vi "align set.vi"(8 "error in (no error)":errorcluster, 11 "align position":T1) -> (0 "error out":errorcluster, 1 "position out":cluster{"X":dbl, "y":dbl, "degree":dbl})   [LabVIEW 2019]
uses:
  align position.ctl
  subVI/move/position cluster.ctl
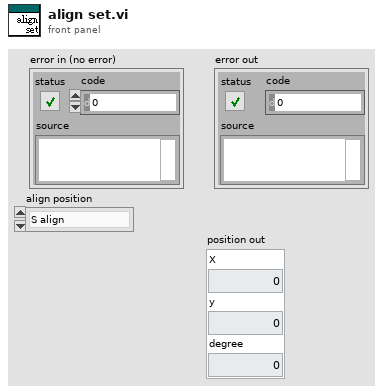
[diagram p1: front panel]
types:
  T1 = typedef "align position.ctl" = enum16{"S align", "vision align", "box align", "box to room align"}
  T2 = typedef "position cluster.ctl" = cluster{"X":dbl, "Y":dbl, "Angle":dbl}
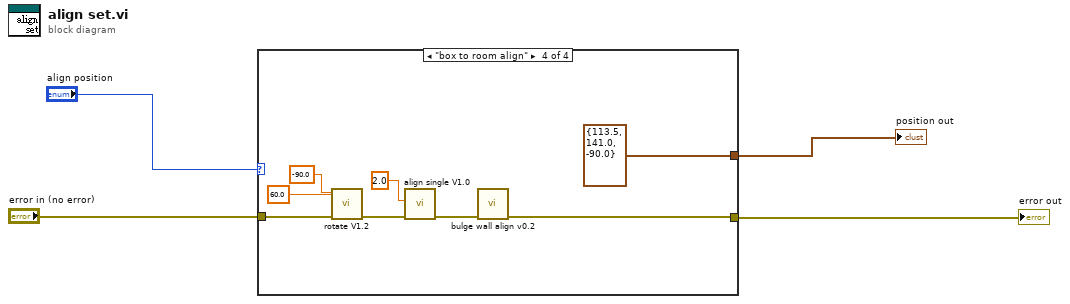
[diagram p0: block diagram]
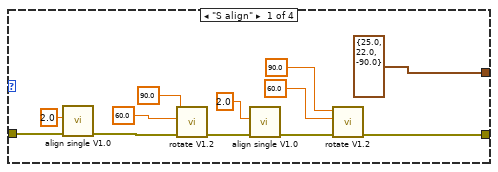
[diagram p2: hidden frame]
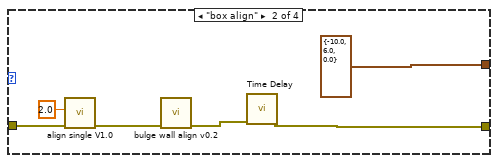
[diagram p3: hidden frame]
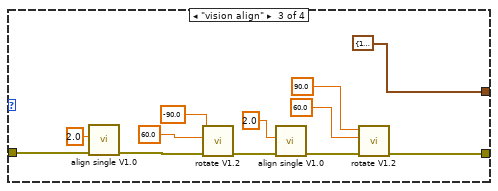
[diagram p4: hidden frame]
diagram:
  n1 = case shown="\"box to room align\"" "align position" {
    tunnel: "error in (no error)" -> [w16 w20 w25 w40]
    tunnel: [w15 w17 w24 w35] -> w3
    tunnel: [cluster{"x":dbl, "y":dbl, "degree":dbl} {"x"=25.0, "y"=22.0, "degree"=-90.0} ("position out") T2 {"X"=-10.0, "Y"=6.0, "Angle"=0.0} ("position out") cluster{"x":dbl, "y":dbl, "degree":dbl} {"x"=103.0, "y"=178.0, "degree"=0.0} ("position out") T2 {"X"=113.5, "Y"=141.0, "Angle"=-90.0} ("position out")] -> w1
    frame "S align" {
      n2 = call "align single V1.0.vi"("error in (no error)"=w16, "Target (Volt)"=2.0) -> ("error out"=w12:errorcluster)  [unwired: 9 in]
      n3 = call "rotate V1.2.vi"("error in (no error)"=w12, "speed"=60.0, "degree"=90.0) -> ("error out"=w11:errorcluster)  [unwired: 8 in]
      n4 = call "align single V1.0.vi"("error in (no error)"=w11, "Target (Volt)"=2.0) -> ("error out"=w10:errorcluster)  [unwired: 9 in]
      n5 = call "rotate V1.2.vi"("error in (no error)"=w10, "speed"=60.0, "degree"=90.0) -> ("error out"=w15:errorcluster)  [unwired: 8 in]
    }
    frame "box align" {
      n6 = call "align single V1.0.vi"("error in (no error)"=w20, "Target (Volt)"=2.0) -> ("error out"=w19:errorcluster)  [unwired: 9 in]
      n7 = call "bulge wall align v0.2.vi"("Error In"=w19) -> ("Error Out"=w22:errorcluster)  [unwired: 10 in]
      n8 = call "Time Delay"("error in (no error)"=w22) -> ("error out"=w17:errorcluster)  [unwired: 10 in]
    }
    frame "vision align" {
      n9 = call "align single V1.0.vi"("error in (no error)"=w25, "Target (Volt)"=2.0) -> ("error out"=w32:errorcluster)  [unwired: 9 in]
      n10 = call "rotate V1.2.vi"("error in (no error)"=w32, "speed"=60.0, "degree"=-90.0) -> ("error out"=w31:errorcluster)  [unwired: 8 in]
      n11 = call "align single V1.0.vi"("error in (no error)"=w31, "Target (Volt)"=2.0) -> ("error out"=w30:errorcluster)  [unwired: 9 in]
      n12 = call "rotate V1.2.vi"("error in (no error)"=w30, "speed"=60.0, "degree"=90.0) -> ("error out"=w24:errorcluster)  [unwired: 8 in]
    }
    frame "box to room align" {
      n13 = call "rotate V1.2.vi"("error in (no error)"=w40, "speed"=60.0, "degree"=-90.0) -> ("error out"=w39:errorcluster)  [unwired: 8 in]
      n14 = call "align single V1.0.vi"("error in (no error)"=w39, "Target (Volt)"=2.0) -> ("error out"=w38:errorcluster)  [unwired: 9 in]
      n15 = call "bulge wall align v0.2.vi"("Error In"=w38) -> ("Error Out"=w35:errorcluster)  [unwired: 10 in]
    }
  }
  "error out" <- w3
  "position out" <- w1
